vi "Control Servo.vi"(7 "servo queue":refnum<queue>, 8 "error in (no error)":errorcluster, 9 "setpoint":dbl, 10 "force":dbl, 11 "Controller in":refnum<class "Controller.lvclass">) -> (0 "error out":errorcluster, 2 "servo pw (us)":dbl)   [LabVIEW 2020]
uses:
  Hardware/Actuators/Servos/Servo.lvclass
  Controllers/Controller.lvclass
  Hardware/Actuators/Servos/Servo.lvclass/Servo.ctl
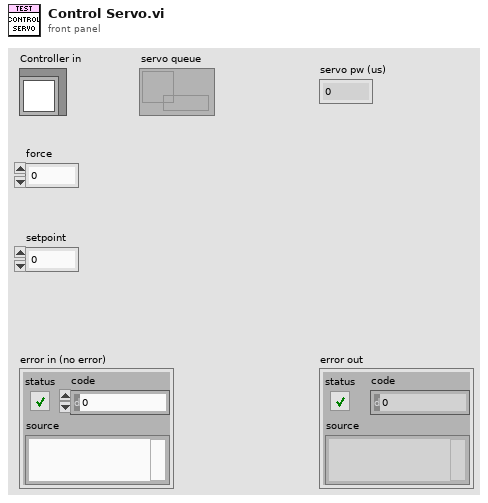
[diagram p1: front panel]
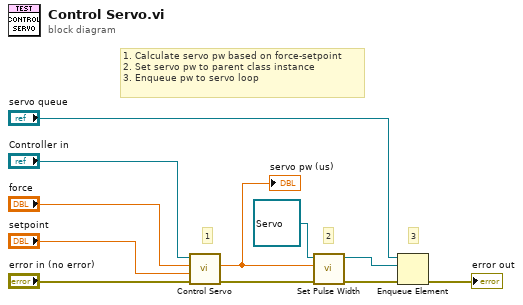
[diagram p0: block diagram]
diagram:
  # "3"
  # "2"
  # "1"
  # "1. Calculate servo pw based on force-setpoint\n2. Set servo pw to parent class instance\n3. Enqueue pw to servo loop"
  n1 = call-dynamic "Control Servo.vi"("error in (no error)"="error in (no error)", "setpoint (V)"="setpoint", "force (V)"="force", "Controller in"="Controller in") -> ("error out"=w7:errorcluster, "servo pw (us)"=w6:dbl)  [unwired: 5 in, 1 out]
  "servo pw (us)" <- w6
  n2 = call "Set Pulse Width.vi"("error in (no error)"=w7, "pulse width (micro-sec)"=w6, "Servo in"=refnum<class "Servo.lvclass"> refnum) -> ("error out"=w8:errorcluster, "Servo out"=w10:refnum<class "Servo.lvclass">)  [unwired: 7 in]
  n3 = Enqueue Element(queue="servo queue", element=w10, error in (no error)=w8) -> (error out=→"error out":errorcluster)  [unwired: 1 in, 2 out]
